vi "Write JSON Config.vi"(6 "Pretty Print?":bool, 8 "error in (no error)":errorcluster, 11 "Concatenate_STR in":refnum<class "Concatenate_STR.lvclass">) -> (0 "error out":errorcluster, 2 "JSON":string, 3 "Concatenate_STR out":refnum<class "Concatenate_STR.lvclass">)   [LabVIEW 2021, in "Concatenate_STR.lvclass"]
uses:
  Concatenate_STR.lvclass
  C:/Program Files (x86)/National Instruments/LabVIEW 2021/vi.lib/TSA/Abstract Data Classes/Abs_Types/Type/Abs_Type.lvclass
  Concatenate_STR.lvclass/Concatenate_STR.ctl
  <vilib>/JDP Science/JSONtext/Make JSON Array.vi
  <vilib>/JDP Science/JSONtext/Merge into Object.vi
  <vilib>/JDP Science/JSONtext/Make JSON Object.vi
  <vilib>/Utility/LVClass/Get LV Class Name.vi
  <vilib>/JDP Science/JSONtext/support/Format JSON Array Text.vi
  <vilib>/JDP Science/JSONtext/support/Format JSON Object.vi
  <vilib>/JDP Science/JSONtext/Get all Object Items.vi
  <vilib>/JDP Science/JSONtext/Set Multiple Object Items.vi
  Abs_Types/Value/Abs_Value.lvclass
  Abs_Types/String/Abs_String.lvclass
  Abs_Types/Type/Abs_Type.lvclass
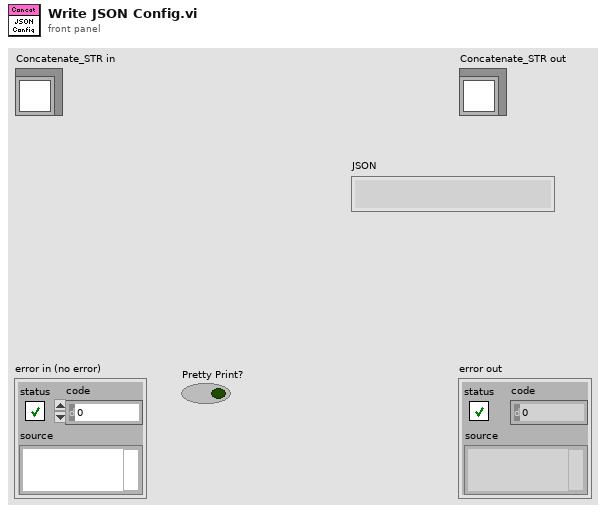
[diagram p1: front panel]
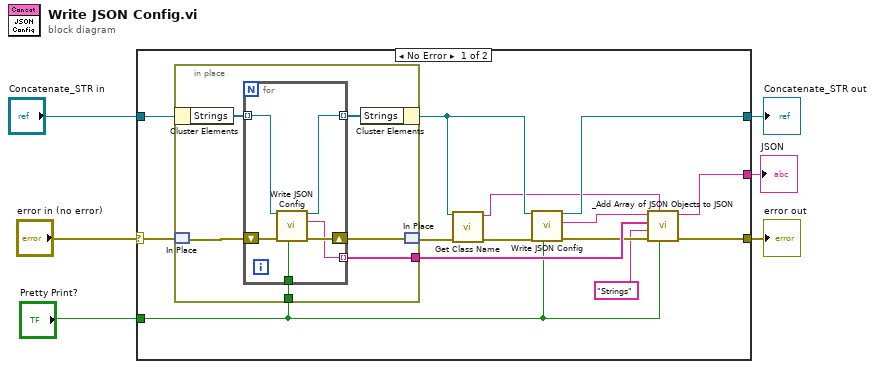
[diagram p0: block diagram]
diagram:
  n1 = case shown="No Error" "error in (no error)" {
    selector: "error in (no error)" -> [w16 w34]
    tunnel: "Concatenate_STR in" -> [w20 w33]
    tunnel: [w19 w33] -> w2
    tunnel: [w12 _] -> w3
    tunnel: [w11 w34] -> w1
    tunnel: "Pretty Print?" -> [w10 _]
    frame No Error {
      n2 = in-place {
        in-place-border: w10 -> [w25]
        in-place-border: [w23] -> w18
        n3 = in-place-cluster #1(w20) -> ("Strings"=w22:refnum<class "Abs_Value.lvclass">[])
        n4 = in-place-match #2(w16) -> (w26:errorcluster)
        n5 = for {
          tunnel: w25 -> [w31]
          tunnel: [w29] -> w23 mode=indexing
          tunnel: w22 -> [w28] mode=indexing
          tunnel: [w27] -> w21 mode=indexing
          shift-right: [w30] -> w24
          shift-left: w26 -> [w32]
          n6 = call-dynamic "Write JSON Config.vi"("Pretty Print?"=w31, "error in (no error)"=w32, "Abs_Type in"=w28) -> ("error out"=w30:errorcluster, "JSON"=w29:string, "Abs_Type out"=w27:refnum<class "Abs_Value.lvclass">)  [unwired: 6 in]
        }
        n7 = in-place-cluster #1("Strings"=w21) -> (w14:refnum<class "Concatenate_STR.lvclass">)
        n8 = in-place-match #2(w24) -> (w17:errorcluster)
      }
      n9 = call "Get Class Name.vi"("error in (no error)"=w17, "Abs_Type in"=w14) -> ("error out"=w15:errorcluster, "class name"=w9:string)  [unwired: 8 in]
      n10 = call-parent "Write JSON Config.vi"("Pretty Print?"=w10, "error in (no error)"=w15, "Abs_Type in"=w14) -> ("error out"=w13:errorcluster, "JSON"=w8:string, "Abs_Type out"=w19:refnum<class "Concatenate_STR.lvclass">)  [unwired: 6 in]
      n11 = call "_Add Array of JSON Objects to JSON.vi"("Pretty Print?"=w10, "JSON Object Name"=w9, "error in (no error)"=w13, "JSON Array Name"="Strings", "JSON Objects"=w18, "JSON"=w8) -> ("error out"=w11:errorcluster, "<JSON>"=w12:string)  [unwired: 4 in]
    }
    frame Error {
    }
  }
  "error out" <- w1
  "Concatenate_STR out" <- w2
  "JSON" <- w3
